vi "Read_By_Datatype.vi"(8 "error in (no error)":errorcluster, 9 "Datatype":T1, 10 "offset":i32, 11 "tag handle":i32) -> (0 "error out":errorcluster, 1 "Datatype":T1, 2 "tag value":variant, 3 "tag handle out":i32)   [LabVIEW 2016]
uses:
  Datatype.ctl
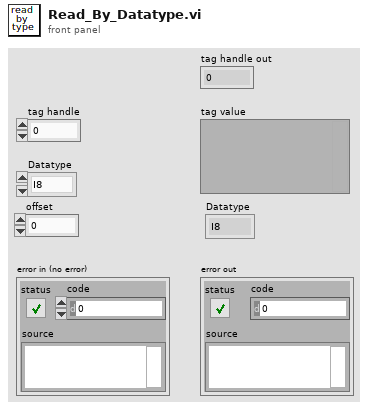
[diagram p1: front panel]
types:
  T1 = typedef "Datatype.ctl" = enum16{"I8", "I16", "I32", "I64", "U8", "U16", "U32", "U64", "FLOAT", "DOUBLE", "BOOL"}
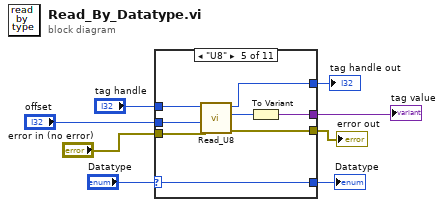
[diagram p0: block diagram]
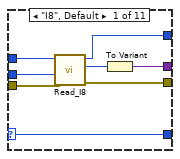
[diagram p2: hidden frame]
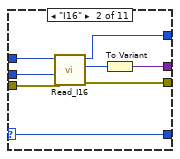
[diagram p3: hidden frame]
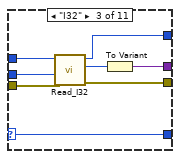
[diagram p4: hidden frame]
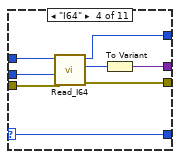
[diagram p5: hidden frame]
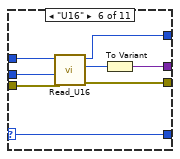
[diagram p6: hidden frame]
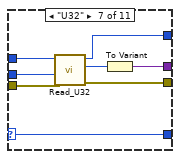
[diagram p7: hidden frame]
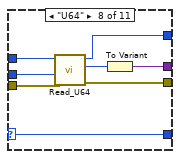
[diagram p8: hidden frame]
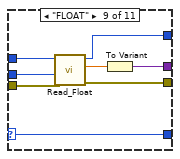
[diagram p9: hidden frame]
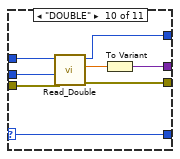
[diagram p10: hidden frame]
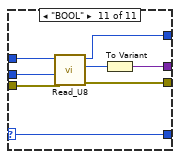
[diagram p11: hidden frame]
diagram:
  n1 = case shown="\"U8\"" "Datatype" {
    selector: "Datatype" -> [w10 w18 w26 w34 w42 w50 w58 w66 w74 w82 w90]
    tunnel: "tag handle" -> [w16 w24 w32 w40 w48 w56 w64 w72 w80 w88 w96]
    tunnel: "error in (no error)" -> [w15 w23 w31 w39 w47 w55 w63 w71 w79 w87 w95]
    tunnel: [w14 w22 w30 w38 w46 w54 w62 w70 w78 w86 w94] -> w6
    tunnel: [w13 w21 w29 w37 w45 w53 w61 w69 w77 w85 w93] -> w7
    tunnel: [w11 w19 w27 w35 w43 w51 w59 w67 w75 w83 w91] -> w8
    tunnel: [w10 w18 w26 w34 w42 w50 w58 w66 w74 w82 w90] -> w2
    tunnel: "offset" -> [w9 w17 w25 w33 w41 w49 w57 w65 w73 w81 w89]
    frame "I8", Default {
      n2 = call "Read_I8.vi"("error in (no error)"=w15, "offset"=w9, "tag handle"=w16) -> ("error out"=w14:errorcluster, "tag value"=w12:i8, "tag handle out"=w13:i32)  [unwired: 6 in]
      n3 = To Variant(anything=w12) -> (Variant=w11:variant)
    }
    frame "I16" {
      n4 = call "Read_I16.vi"("error in (no error)"=w23, "offset"=w17, "tag handle"=w24) -> ("error out"=w22:errorcluster, "tag value"=w20:i16, "tag handle out"=w21:i32)  [unwired: 6 in]
      n5 = To Variant(anything=w20) -> (Variant=w19:variant)
    }
    frame "I32" {
      n6 = call "Read_I32.vi"("error in (no error)"=w31, "offset"=w25, "tag handle"=w32) -> ("error out"=w30:errorcluster, "tag value"=w28:i32, "tag handle out"=w29:i32)  [unwired: 6 in]
      n7 = To Variant(anything=w28) -> (Variant=w27:variant)
    }
    frame "I64" {
      n8 = call "Read_I64.vi"("error in (no error)"=w39, "offset"=w33, "tag handle"=w40) -> ("error out"=w38:errorcluster, "tag value"=w36:i64, "tag handle out"=w37:i32)  [unwired: 6 in]
      n9 = To Variant(anything=w36) -> (Variant=w35:variant)
    }
    frame "U8" {
      n10 = call "Read_U8.vi"("error in (no error)"=w47, "offset"=w41, "tag handle"=w48) -> ("error out"=w46:errorcluster, "tag value"=w44:u8, "tag handle out"=w45:i32)  [unwired: 6 in]
      n11 = To Variant(anything=w44) -> (Variant=w43:variant)
    }
    frame "U16" {
      n12 = call "Read_U16.vi"("error in (no error)"=w55, "offset"=w49, "tag handle"=w56) -> ("error out"=w54:errorcluster, "tag value"=w52:u16, "tag handle out"=w53:i32)  [unwired: 6 in]
      n13 = To Variant(anything=w52) -> (Variant=w51:variant)
    }
    frame "U32" {
      n14 = call "Read_U32.vi"("error in (no error)"=w63, "offset"=w57, "tag handle"=w64) -> ("error out"=w62:errorcluster, "tag value"=w60:u32, "tag handle out"=w61:i32)  [unwired: 6 in]
      n15 = To Variant(anything=w60) -> (Variant=w59:variant)
    }
    frame "U64" {
      n16 = call "Read_U64.vi"("error in (no error)"=w71, "offset"=w65, "tag handle"=w72) -> ("error out"=w70:errorcluster, "tag value"=w68:u64, "tag handle out"=w69:i32)  [unwired: 6 in]
      n17 = To Variant(anything=w68) -> (Variant=w67:variant)
    }
    frame "FLOAT" {
      n18 = call "Read_Float.vi"("error in (no error)"=w79, "offset"=w73, "tag handle"=w80) -> ("error out"=w78:errorcluster, "tag value"=w76:sgl, "tag handle out"=w77:i32)  [unwired: 6 in]
      n19 = To Variant(anything=w76) -> (Variant=w75:variant)
    }
    frame "DOUBLE" {
      n20 = call "Read_Double.vi"("error in (no error)"=w87, "offset"=w81, "tag handle"=w88) -> ("error out"=w86:errorcluster, "tag value"=w84:dbl, "tag handle out"=w85:i32)  [unwired: 6 in]
      n21 = To Variant(anything=w84) -> (Variant=w83:variant)
    }
    frame "BOOL" {
      n22 = call "Read_U8.vi"("error in (no error)"=w95, "offset"=w89, "tag handle"=w96) -> ("error out"=w94:errorcluster, "tag value"=w92:u8, "tag handle out"=w93:i32)  [unwired: 6 in]
      n23 = To Variant(anything=w92) -> (Variant=w91:variant)
    }
  }
  "error out" <- w6
  "tag handle out" <- w7
  "tag value" <- w8
  "Datatype" <- w2
